vi "Pose2DtoVector.vi"(9 "Tail":T2, 11 "Nose":T2) -> (3 "Vector":T1)   [LabVIEW 2018]
uses:
  Pose2D.ctl
  Vector/Vector2D.ctl
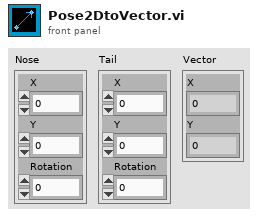
[diagram p1: front panel]
types:
  T1 = typedef "Vector2D.ctl" = cluster{"X":dbl, "Y":dbl}
  T2 = typedef "Pose2D.ctl" = cluster{"X":dbl, "Y":dbl, "Rotation":dbl}
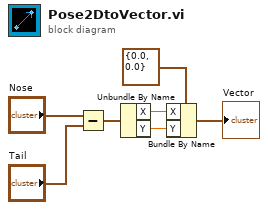
[diagram p0: block diagram]
diagram:
  n1 = Subtract(x="Nose", y="Tail") -> (x-y=w5:T2)
  n2 = Unbundle By Name(w5) -> ("X"=w3:dbl, "Y"=w2:dbl)
  n3 = Bundle By Name(cluster=T1 {"X"=0.0, "Y"=0.0} ("Vector 2"), "X"=w3, "Y"=w2) -> (→"Vector":T1)
